vi "C867_Send_Command.vi"(8 "entrée d'erreur (pas d'erreur)":errorcluster, 10 "szCommand":string="SVO 1 1", 11 "ID en entrée":i32) -> (0 "sortie d'erreur":errorcluster, 2 "szCommand out":string, 3 "ID en sortie":i32)   [LabVIEW 2026]
uses:
  C867-VIs/Low Level/PI_GCS2_DLL_x64.dll
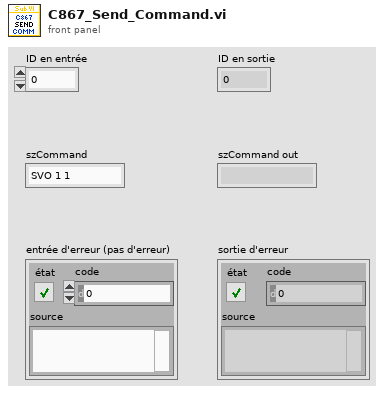
[diagram p1: front panel]
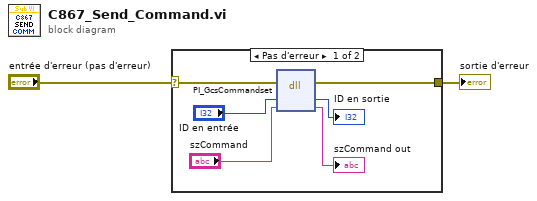
[diagram p0: block diagram]
diagram:
  n1 = case shown="Pas d'erreur" "entrée d'erreur (pas d'erreur)" {
    selector: "entrée d'erreur (pas d'erreur)" -> [w5 w9]
    tunnel: [w8 w9] -> w2
    frame No Error {
      n2 = dll-call lib="C:/Users/Sebastien/Documents/GitHub/LABVIEW-Useful-codes/Device_control/PC-C867-IO Control/v0.1/SubVI/PI-C867/C867-VIs/Low Level/PI_GCS2_DLL_x64.dll" fn="PI_GcsCommandset"(error in=w5, "ID"="ID en entrée", "szCommand"="szCommand") -> (error out=w8:errorcluster, "ID"=→"ID en sortie":i32, "szCommand"=→"szCommand out":string)  [unwired: 3 in, 1 out]
    }
    frame Error {
    }
  }
  "sortie d'erreur" <- w2
